vi "PicoScope4000aGetAnalogueOffset.vi"(8 "error in (no error)":errorcluster, 9 "Coupling":i16(ring)=1 items=["AC", "DC"], 10 "Range":u16(ring)=4000 items=["10mV"=0, "20mV"=1, "50mV"=2, "100mV"=3, "200mV"=4, "500mV"=5, "1V"=6, "2V"=7, "5V"=8, "10V"=9, "20V"=10, "50V"=11, "100V"=12, "200V"=13, "1KV_2_5V"=6003, "1KV_5V"=6004, "1KV_12_5V"=6005, "1KV_25V"=6006, "1KV_50V"=6007, "1KV_125V"=6008, "1KV_250V"=6009, "1KV_500V"=6010, "1KV_1000V"=6011, "CURRENT_CLAMP_200A_2kA_1A"=4000, "CURRENT_CLAMP_200A_2kA_2A"=4001, "CURRENT_CLAMP_200A_2kA_5A"=4002, "CURRENT_CLAMP_200A_2kA_10A"=4003, "CURRENT_CLAMP_200A_2kA_20A"=4004, "CURRENT_CLAMP_200A_2kA_50A"=4005, "CURRENT_CLAMP_200A_2kA_100A"=4006, "CURRENT_CLAMP_200A_2kA_200A"=4007, "CURRENT_CLAMP_200A_2kA_500A"=4008, "CURRENT_CLAMP_200A_2kA_1000A"=4009, "CURRENT_CLAMP_200A_2kA_2000A"=4010, "CURRENT_CLAMP_40A_100mA"=5000, "CURRENT_CLAMP_40A_200mA"=5001, "CURRENT_CLAMP_40A_500mA"=5002, "CURRENT_CLAMP_40A_1A"=5003, "CURRENT_CLAMP_40A_2A"=5004, "CURRENT_CLAMP_40A_5A"=5005, "CURRENT_CLAMP_40A_10A"=5006, "CURRENT_CLAMP_40A_20A"=5007, "CURRENT_CLAMP_40A_40A"=5008, "CURRENT_CLAMP_2000ARMS_10A"=6500, "CURRENT_CLAMP_2000ARMS_20A"=6501, "CURRENT_CLAMP_2000ARMS_50A"=6502, "CURRENT_CLAMP_2000ARMS_100A"=6503, "CURRENT_CLAMP_2000ARMS_200A"=6504, "CURRENT_CLAMP_2000ARMS_500A"=6505, "CURRENT_CLAMP_2000ARMS_1000A"=6506, "CURRENT_CLAMP_2000ARMS_2000A"=6507, "CURRENT_CLAMP_2000ARMS_5000A"=6508, "x10_Probe_100mV"=32, "x10_Probe_200mV"=33, "x10_Probe_500mV"=34, "x10_Probe_1V"=35, "x10_Probe_2V"=36, "x10_Probe_5V"=37, "x10_Probe_10V"=38, "x10_Probe_20V"=39, "x10_Probe_50V"=40, "x10_Probe_100V"=41, "x10_Probe_200V"=42, "x10_Probe_500V"=43, "CURRENT_CLAMP_60A_2A"=10500, "CURRENT_CLAMP_60A_5A"=10501, "CURRENT_CLAMP_60A_10A"=10502, "CURRENT_CLAMP_60A_20A"=10503, "CURRENT_CLAMP_60A_50A"=10504, "CURRENT_CLAMP_60A_60A"=10505, "CURRENT_CLAMP_60A_V2_0_5A"=10600, "CURRENT_CLAMP_60A_V2_1A"=10601, "CURRENT_CLAMP_60A_V2_2A"=10602, "CURRENT_CLAMP_60A_V2_5A"=10603, "CURRENT_CLAMP_60A_V2_10A"=10604, "CURRENT_CLAMP_60A_V2_20A"=10605, "CURRENT_CLAMP_60A_V2_50A"=10606, "CURRENT_CLAMP_60A_V2_60A"=10607, "RESISTANCE_LEAD_NEG5_TO_20OHM"=7000, "RESISTANCE_LEAD_NEG50_TO_200OHM"=7001, "RESISTANCE_LEAD_NEG500_TO_2KOHM"=7002, "RESISTANCE_LEAD_NEG5K_TO_20KOHM"=7003, "RESISTANCE_LEAD_NEG50K_TO_LEAD_200KOHM"=7004, "RESISTANCE_LEAD_NEG500K_TO_LEAD_2MOHM"=7005, "RESISTANCE_LEAD_DIODE_TEST"=7006, "HT_NEG3_TO_5KV"=8950, "HT_NEG3_TO_10KV"=8951, "HT_NEG5_TO_20KV"=8952, "HT_NEG5_TO_50KV"=8953, "HT_NEG5_TO_100KV"=8954, "HT_NEG3_TO_5KV_INVERTED"=8955, "HT_NEG3_TO_10KV_INVERTED"=8956, "HT_NEG5_TO_20KV_INVERTED"=8957, "HT_NEG5_TO_50KV_INVERTED"=8958, "HT_NEG5_TO_100KV_INVERTED"=8959, "TEMPERATURE_NEG50_TO_150DEGC"=9000, "PRESSURE_SENSOR_-100k-150k_PASCALS"=9100, "PRESSURE_SENSOR_-100k_TO_400k_PASCALS"=9101, "PRESSURE_SENSOR_-200k_TO_800k_PASCALS"=9102, "PRESSURE_SENSOR_-400k_TO_1600k_PASCALS"=9103, "PRESSURE_SENSOR_-400k_TO_3400k_PASCALS"=9104, "PRESSURE_SENSOR_-150k_TO_1350k_PASCALS"=9105], 11 "handle in":i16) -> (0 "error out":errorcluster, 1 "minimumValue":sgl, 2 "maximumValue":sgl, 3 "handle out":i16)   [LabVIEW 2010]
doc: "Calls GetAnalogueOffset"
uses:
  Program Files/Pico Technology/SDK/lib/ps4000a.dll
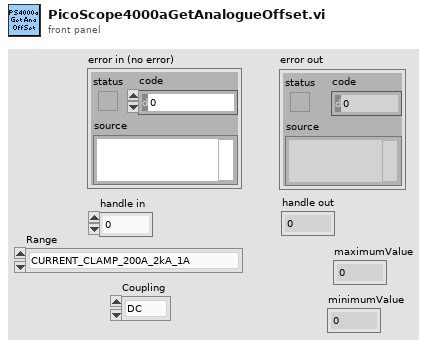
[diagram p1: front panel]
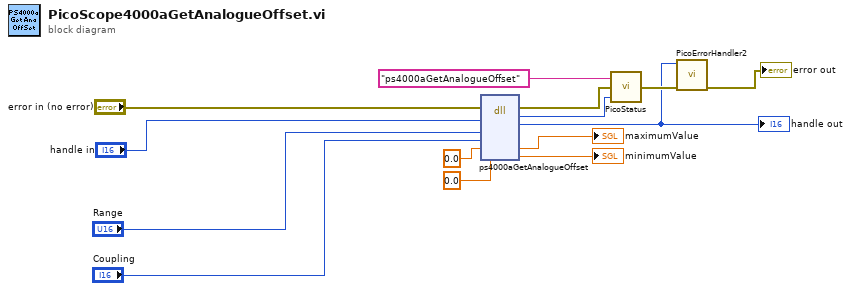
[diagram p0: block diagram]
diagram:
  n1 = dll-call lib="/Program Files/Pico Technology/SDK/lib/ps4000a.dll" fn="ps4000aGetAnalogueOffset" ("ps3000.dll:_ps3000_open_unit@0")(error in="error in (no error)", "handle"="handle in", "range"="Range", "coupling"="Coupling", "maximumVoltage"=sgl 0.0, "minimumVoltage"=sgl 0.0) -> (error out=w5:errorcluster, "PICO_STATUS"=w3:u32, "handle"=w2:i16, "maximumVoltage"=→"maximumValue":sgl, "minimumVoltage"=→"minimumValue":sgl)  [unwired: 4 in, 1 out]
  "handle out" <- w2
  n2 = call "PicoStatus.vi"("PICO STATUS"=w3, "error in"=w5, "source"="ps4000aGetAnalogueOffset") -> ("error out"=w6:errorcluster)
  n3 = call "PicoErrorHandler2.vi"("error in (no error)"=w6, "handle In"=w2) -> ("error out"=→"error out":errorcluster)  [unwired: 9 in]
